vi "Test Shared Resource Location.vi"(8 "error in":errorcluster) -> (0 "error out":errorcluster)   [LabVIEW 2019]
uses:
  Setting Database/Setting Database.lvclass
  C:/Program Files (x86)/National Instruments/LabVIEW 2019/vi.lib/JKI/JKI SMO/SMO/SMO.lvclass
  <vilib>/JKI/JKI SMO/SMO/SMO.lvclass
  <vilib>/addons/_JKI Toolkits/Caraya/classes/Assert/Assert True.vi
  <vilib>/addons/_JKI Toolkits/Caraya/classes/Test/Test.lvclass
  <vilib>/addons/_JKI Toolkits/Caraya/classes/Assert/Assert.lvclass
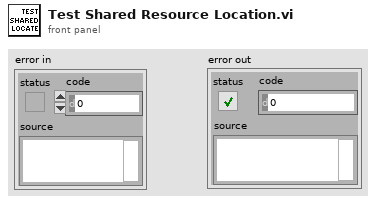
[diagram p1: front panel]
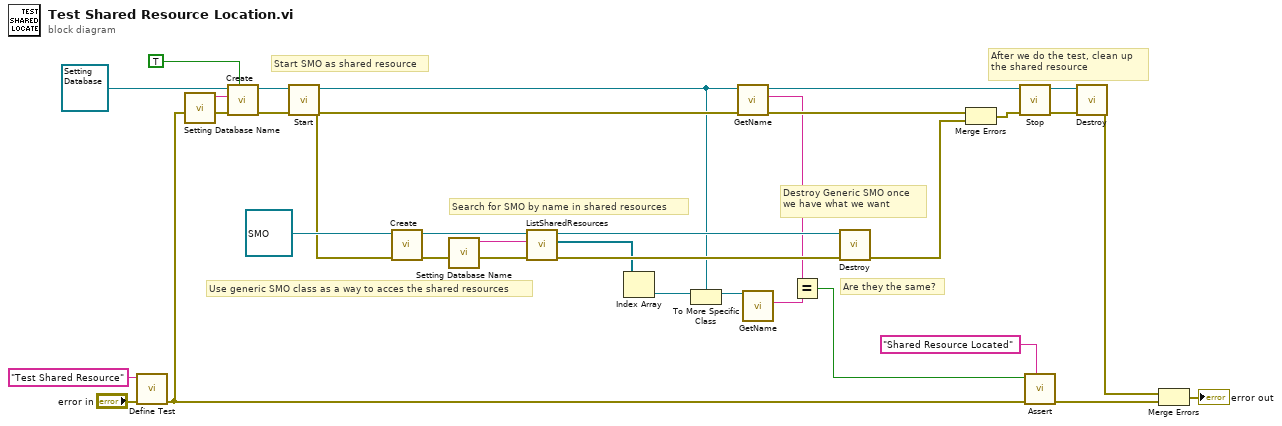
[diagram p0: block diagram]
diagram:
  # "After we do the test, clean up the shared resource"
  # "Destroy Generic SMO once we have what we want"
  # "Are they the same?"
  # "Search for SMO by name in shared resources"
  # "Use generic SMO class as a way to acces the shared resources"
  # "Start SMO as shared resource"
  n1 = call <vilib>:"Define Test.vi"("error in (no error)"="error in", "Label (VI Title)"="Test Shared Resource") -> ("error out"=w24:errorcluster)  [unwired: 8 in, 1 out]
  n2 = call "Setting Database Name.vi"("error in (no error)"=w24) -> ("error out"=w25:errorcluster, "Name"=w15:string)  [unwired: 9 in]
  n3 = call <vilib>:"Create.vi"("Shared Resource (F)"=TRUE, "error in (no error)"=w25, "Subsystem Name (optional)"=w15, "SMO"=refnum<class "Setting Database.lvclass"> refnum ("Setting Database.lvclass")) -> ("error out"=w32:errorcluster, "SMO out"=w20:refnum<class "Setting Database.lvclass">)  [unwired: 5 in, 1 out]
  n4 = call <vilib>:"Start.vi"("error in (no error)"=w32, "SMO"=w20) -> ("error out"=w7:errorcluster, "SMO out"=w4:refnum<class "Setting Database.lvclass">)  [unwired: 8 in]
  n5 = call <vilib>:"Create.vi"("error in (no error)"=w7, "SMO"=refnum<class "SMO.lvclass"> refnum) -> ("error out"=w23:errorcluster, "SMO out"=w17:refnum<class "SMO.lvclass">)  [unwired: 7 in, 1 out]
  n6 = call "Setting Database Name.vi"("error in (no error)"=w23) -> ("error out"=w22:errorcluster, "Name"=w13:string)  [unwired: 9 in]
  n7 = call <vilib>:"ListSharedResources.vi"("error in (no error)"=w22, "Filter (regex|name)"=w13, "SMO in"=w17) -> ("error out"=w30:errorcluster, "Shared Resources"=w8:refnum<class "SMO.lvclass">[], "SMO out"=w12:refnum<class "SMO.lvclass">)  [unwired: 5 in, 1 out]
  n8 = Index Array(array=w8) -> (element=w11:refnum<class "SMO.lvclass">)  [unwired: 1 in]
  n9 = To More Specific Class(target class=w4, reference=w11) -> (specific class reference=w2:refnum<class "Setting Database.lvclass">)  [unwired: 1 in, 1 out]
  n10 = call <vilib>:"GetName.vi"("error in (no error)"=w7, "SMO"=w4) -> ("error out"=w6:errorcluster, "Name"=w3:string, "SMO out"=w5:refnum<class "Setting Database.lvclass">)  [unwired: 6 in, 1 out]
  n11 = call <vilib>:"GetName.vi"("SMO"=w2) -> ("Name"=w1:string)  [unwired: 7 in, 3 out]
  n12 = Equal?(x=w3, y=w1) -> (x = y?=w9:bool)
  n13 = call <vilib>:"Destroy.vi"("error in (no error)"=w30, "SMO"=w12) -> ("error out"=w31:errorcluster)  [unwired: 9 in]
  n14 = Merge Errors(w6, w31) -> (w29:errorcluster)
  n15 = call <vilib>:"Stop.vi"("error in (no error)"=w29, "SMO"=w5) -> ("error out"=w33:errorcluster, "SMO out"=w14:refnum<class "Setting Database.lvclass">)  [unwired: 8 in]
  n16 = call-poly <vilib>:"Assert.vi"("Label"="Shared Resource Located" ("Label (VI Title)"), "error in (no error)"=w24, "True?"=w9) -> ("error out"=w34:errorcluster)  [unwired: 7 in, 1 out]
  n17 = call <vilib>:"Destroy.vi"("error in (no error)"=w33, "SMO"=w14) -> ("error out"=w28:errorcluster)  [unwired: 9 in]
  n18 = Merge Errors(w28, w34) -> (→"error out":errorcluster)
